vi "DSF.Shared.Configuration.Framework.Get Custom Parameters.vi"(8 "error in (no error)":errorcluster, 11 "Framework Configuration in":refnum<class "DSF.Shared.Configuration.Framework.lvclass">) -> (0 "error out":errorcluster, 2 "Custom Parameters":variant, 3 "Framework Configuration out":refnum<class "DSF.Shared.Configuration.Framework.lvclass">)   [LabVIEW 2016, in "DSF.Shared.lvlib" / "DSF.Shared.Configuration.Framework.lvclass"]
uses:
  DSF.Shared.Configuration.Framework.lvclass
  DSF.Shared.Configuration.Framework.lvclass/DSF.Shared.Configuration.Framework.ctl
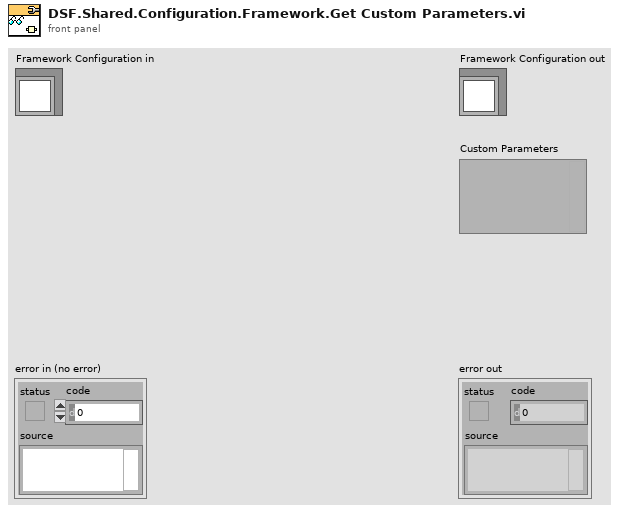
[diagram p1: front panel]
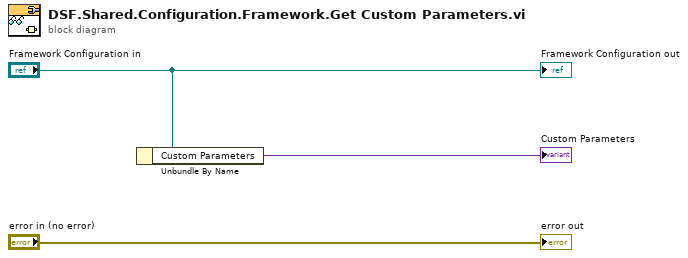
[diagram p0: block diagram]
diagram:
  n1 = Unbundle By Name("Framework Configuration in") -> ("Custom Parameters"=→"Custom Parameters":variant)
  "error out" <- "error in (no error)"
  "Framework Configuration out" <- "Framework Configuration in"
